vi "kinematics.vi"() -> ()   [LabVIEW 2020]
panel:
  in  "정지":bool
  out "Bkt angle(deg)":dbl
  out "Arm angle(deg)":dbl
  out "Boom angle(deg)":dbl
  out "transformation matrix":dbl[][](array[numeric])
  out "gamma_deg":dbl
  out "beta_deg":dbl
  out "alpha_deg":dbl
  in  "Bkt offset(mm)":dbl
  in  "Arm offset(mm)":dbl
  in  "Boom offset(mm)":dbl
  in  "Bucket stroke(mm)":dbl
  in  "Arm stroke(mm)":dbl
  in  "Boom stroke(mm)":dbl
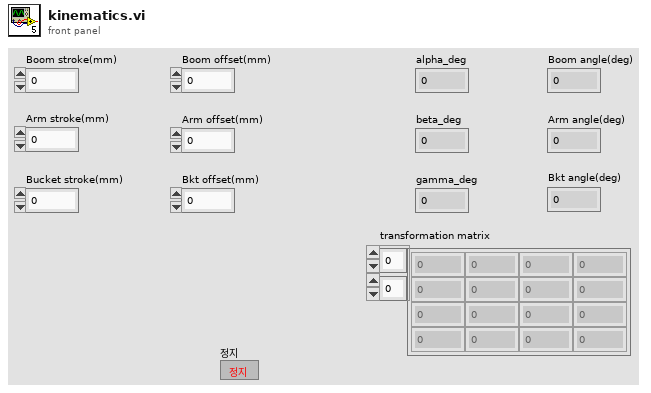
[diagram p1: front panel]
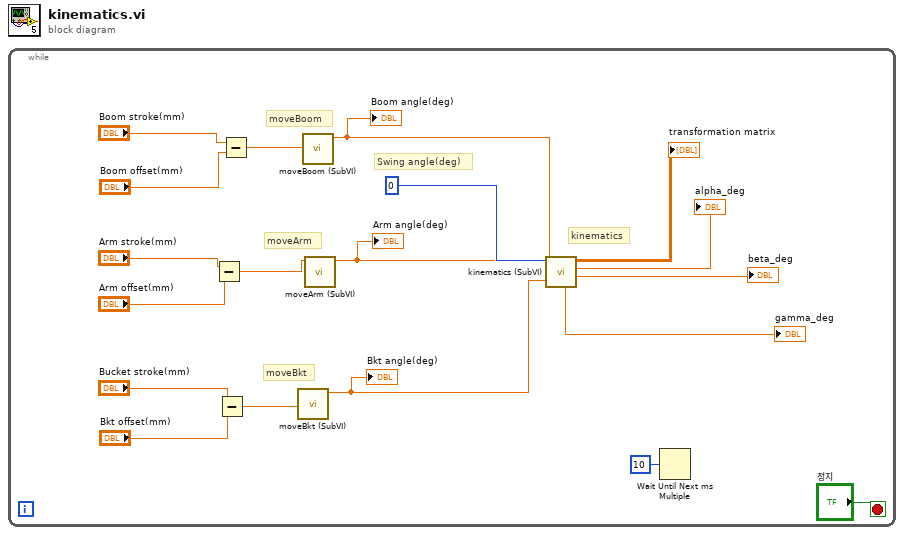
[diagram p0: block diagram]
diagram:
  n1 = while {
    stop <- "정지" stop-if-true
    # "Swing angle(deg)"
    # "kinematics"
    # "moveBkt"
    # "moveArm"
    # "moveBoom"
    n2 = Subtract(x="Arm stroke(mm)", y="Arm offset(mm)") -> (x-y=w12:dbl)
    n3 = Subtract(x="Bucket stroke(mm)", y="Bkt offset(mm)") -> (x-y=w11:dbl)
    n4 = Subtract(x="Boom stroke(mm)", y="Boom offset(mm)") -> (x-y=w13:dbl)
    n5 = call "moveBkt (SubVI).vi"("Bkt stroke(mm)"=w11) -> ("bkt angle(deg)"=w3:sgl)  [unwired: 10 in]
    "Bkt angle(deg)" <- w3
    n6 = call "moveBoom (SubVI).vi"("Boom stoke(mm)"=w13) -> ("Boom angle(deg)"=w5:sgl)  [unwired: 10 in]
    "Boom angle(deg)" <- w5
    n7 = call "moveArm (SubVI).vi"("Arm stoke(mm)"=w12) -> ("Arm angle(deg)"=w4:sgl)  [unwired: 10 in]
    "Arm angle(deg)" <- w4
    n8 = call "kinematics (SubVI).vi"("Bkt angle(deg)"=w3, "Arm angle(deg)"=w4, "Boom angle(deg)"=w5, "Swing angle(deg)"=0) -> ("beta_deg"=→"beta_deg":dbl, "alpha_deg"=→"alpha_deg":dbl, "T"=→"transformation matrix":dbl[][], "gamma_deg"=→"gamma_deg":dbl)  [unwired: 4 in]
    n9 = Wait Until Next ms Multiple(millisecond multiple=u32 10 ("ms 배수")) -> ()  [unwired: 1 out]
  }
